vi "AMC e.bloxx Example - Write Analog Value.vi"() -> ()   [LabVIEW 2013]
doc: "<B>AMC - Analytik & Messtechnik GmbH Chemnitz</B>\n\nLabVIEW Drivers for e.bloxx series from Gantner Instruments\n\nThis example demonstrates the usage of the e.bloxx VIs. You must select your serial settings according to the e.bloxx configuration set via ICP software. Then choose your designated module by Module Address and your variable by Channel. The slider allows you to easily change your desired analog output value."
uses:
  AMC e.bloxx Write Value - Double.vi
panel:
  in  "Value":dbl(slide) scale=0.0..10.0
  out "error out":errorcluster
  in  "stop":bool
  in  "Channel":i32
  in  "Module Address":i32=2
  in  "Parity":enum16{"None", "Odd", "Even", "Mark", "Space"}(ring)=enum."Even"
  in  "Baudrate":u32=115200
  in  "VISA Resource Name":refnum<visa-resource-name>="COM2"
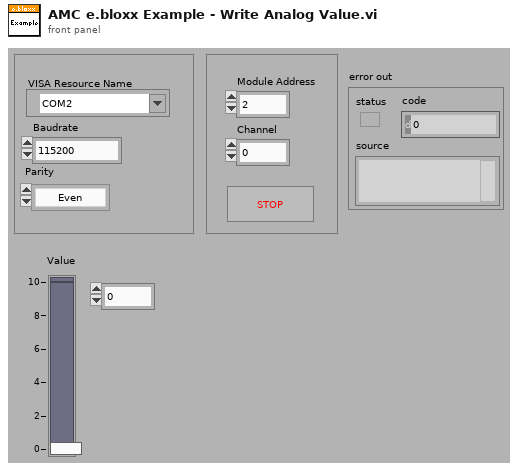
[diagram p1: front panel]
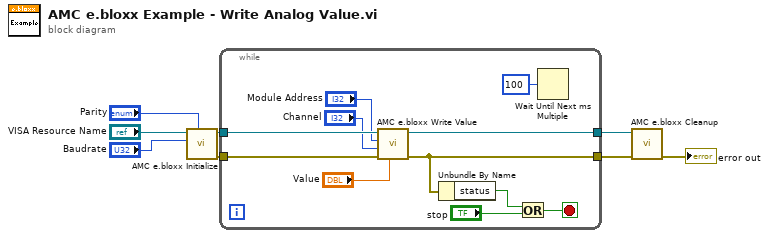
[diagram p0: block diagram]
diagram:
  n1 = call "AMC e.bloxx Initialize.vi"("parity (0:none)"="Parity", "baud rate (9600)"="Baudrate", "VISA resource name"="VISA Resource Name") -> ("error out"=w4:errorcluster, "VISA resource name out"=w5:refnum<visa-resource-name>)  [unwired: 7 in]
  n2 = while {
    tunnel: w5 -> [w19]
    tunnel: w4 -> [w18]
    tunnel: [w12] -> w3
    tunnel: [w11] -> w2
    stop <- w15 stop-if-true
    n3 = call-poly "AMC e.bloxx Write Value.vi"("Value"="Value", "error in (no error)"=w18, "Channel"="Channel", "Module Address"="Module Address", "VISA Resource Name"=w19) -> ("error out"=w11:errorcluster, "VISA Resource Name out"=w12:refnum<visa-resource-name>)  [unwired: 5 in]
    n4 = Unbundle By Name(w11) -> ("status"=w13:bool)
    n5 = Or(x=w13, y="stop") -> (x .or. y?=w15:bool)
    n6 = Wait Until Next ms Multiple(millisecond multiple=u32 100) -> ()  [unwired: 1 out]
  }
  n7 = call "AMC e.bloxx Cleanup.vi"("error in (no error)"=w2, "VISA resource name"=w3) -> ("error out"=→"error out":errorcluster)  [unwired: 9 in]
